vi "PaneZero.vi"(9 "error in (no error)":errorcluster, 10 "Pane":refnum<vi>) -> (1 "error out":errorcluster)   [LabVIEW 2020]
doc: "Set Pane zero to 0,0"
uses:
  <vilib>/Utility/miscctls.llb/LVPointTypeDef.ctl
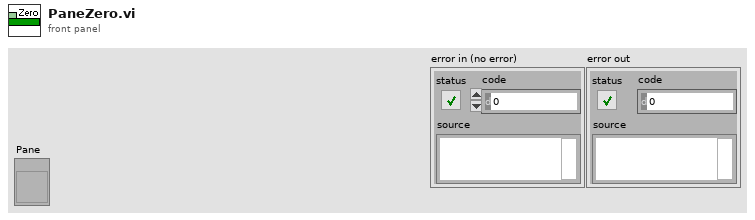
[diagram p1: front panel]
types:
  T1 = typedef "LVPointTypeDef.ctl" = cluster{"Horizontal":i16, "Vertical":i16}
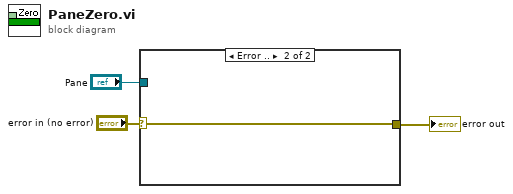
[diagram p0: block diagram]
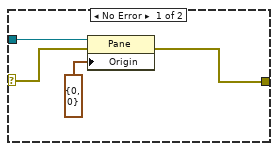
[diagram p2: hidden frame]
diagram:
  n1 = case shown="Error .." "error in (no error)" {
    selector: "error in (no error)" -> [w4 w8]
    tunnel: "Pane" -> [w6 _]
    tunnel: [w5 w8] -> w2
    frame No Error {
      n2 = property class="Pane"(reference=w6, error in=w4, "Origin"=T1 {"Horizontal"=0, "Vertical"=0}) -> (error out=w5:errorcluster)  [unwired: 1 out]
    }
    frame Error {
    }
  }
  "error out" <- w2
